vi "FlowPopup.vi"(11 "Path":path) -> ()   [LabVIEW 2013, in "main.lvlib"]
uses:
  main.lvlib
panel:
  out "Max amplitude 2":dbl
  out "Descending 2":dbl
  out "Ascending 2":dbl
  out "Max amplitude":dbl
  out "Descending":dbl
  out "Ascending":dbl
  in  "Cancel Button":bool
  out "RedGraph":T1(graph)
  out "BlueGraph":T1(graph)
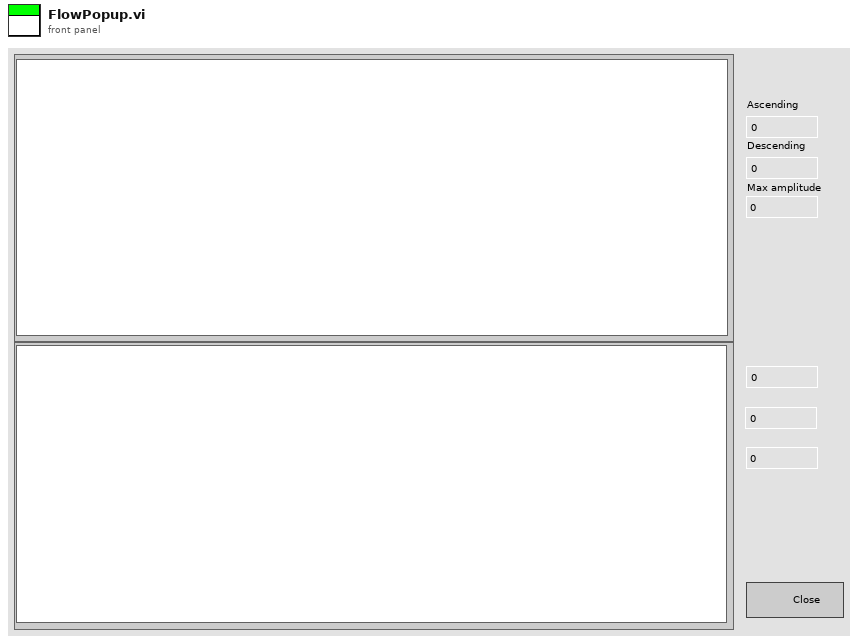
[diagram p1: front panel]
types:
  T1 = cluster{"Array out":dbl[], "Best Linear Fit":dbl[]}[]
  T2 = cluster{dbl[], "Best Linear Fit":dbl[], "slope":dbl, dbl[], "Best Linear Fit":dbl[], "slope":dbl}
  T3 = cluster{dbl[], "Best Linear Fit":dbl[], "slope":dbl}
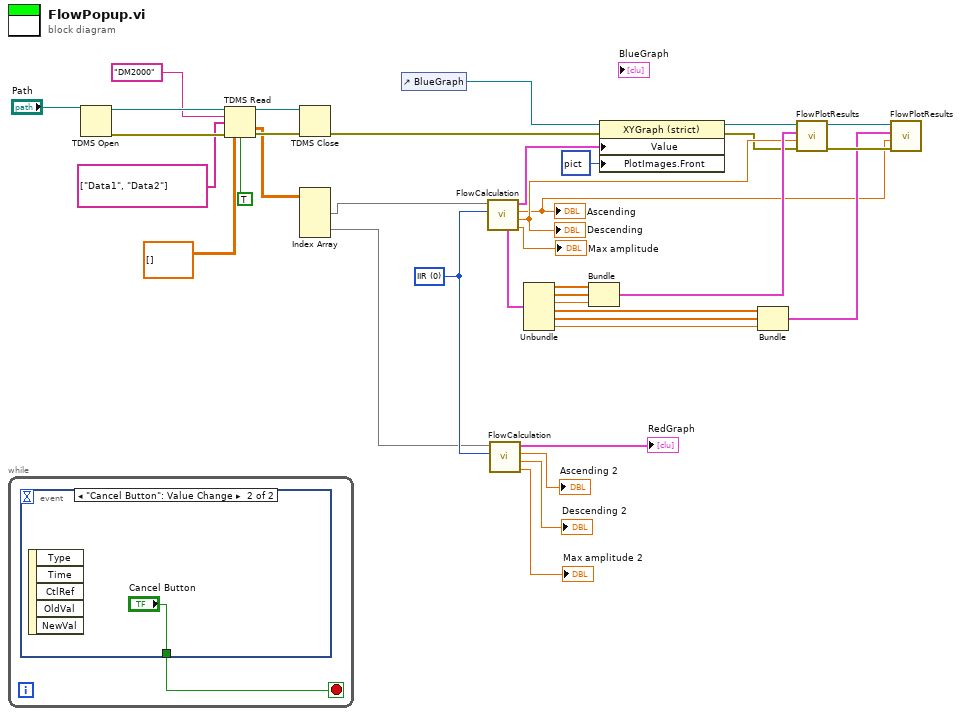
[diagram p0: block diagram]
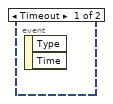
[diagram p2: hidden frame]
diagram:
  w36 = u16 0 items=["IIR", "Butterworth", "None"] ("Filter")
  n1 = while {
    stop <- w38 stop-if-true
    n2 = event shown="[1] \"Cancel Button\": Value Change" {
      selector: _ -> [_ _]
      dyn-events: _ -> [_ _]
      timeout: _ -> [_ _]
      tunnel: [_ "Cancel Button"] -> w38
      event Timeout {
        n3 = event-data() -> ()  [unwired: 1 in, 2 out]
      }
      event "Cancel Button": Value Change {
        n4 = event-data() -> ()  [unwired: 1 in, 5 out]
      }
    }
  }
  n5 = TDMS Open(11:"Path") -> (0:w29:errorcluster, 3:w35:refnum<k34>)  [unwired: 6 in]
  n6 = TDMS Read(0:w35, 5:"DM2000" ("group name in"), 7:string[] ["Data1", "Data2"], 11:w29, 12:dbl[][] [], 13:TRUE ("return channels in file order? (F)")) -> (4:w31:refnum<k34>, 10:w26:dbl[][], 15:w30:errorcluster)  [unwired: 2 in, 3 out]
  n7 = TDMS Close(8:w30, 11:w31) -> (0:w11:errorcluster)  [unwired: 1 out]
  n8 = Index Array(array=w26) -> (element #1=w25:dbl[], element #2=w24:dbl[])  [unwired: 4 in]
  n9 = control-ref of="BlueGraph"() -> (w14:refnum<vi>)
  n10 = call "FlowCalculation.vi"("Filter"=w36, "X"=w25) -> ("Max amplitude"=→"Max amplitude":dbl, "Descending"=w10:dbl, "Ascending"=w3:dbl, "Flow Graph"=w13:T1, "Slopes Out"=w19:T2)  [unwired: 5 in]
  "Ascending" <- w3
  "Descending" <- w10
  n11 = call "FlowCalculation.vi"("Filter"=w36, "X"=w24) -> ("Max amplitude"=→"Max amplitude 2":dbl, "Descending"=→"Descending 2":dbl, "Ascending"=→"Ascending 2":dbl, "Flow Graph"=→"RedGraph":T1)  [unwired: 5 in, 1 out]
  n12 = Unbundle(w19) -> (w18:dbl[], "Best Linear Fit"=w17:dbl[], "slope"=w16:dbl, w7:dbl[], "Best Linear Fit"=w6:dbl[], "slope"=w5:dbl)
  n13 = Bundle(w18, "Best Linear Fit"=w17, "slope"=w16) -> (w15:T3)  [unwired: 1 in]
  n14 = property class="XYGraph (strict)"(reference=w14, error in=w11, "Value"=w13, "PlotImages.Front"=picture data[5B] ("Plot Images:Front")) -> (reference out=w12:refnum<vi>, error out=w2:errorcluster)
  n15 = Bundle(w7, "Best Linear Fit"=w6, "slope"=w5) -> (w4:T3)  [unwired: 1 in]
  n16 = call "FlowPlotResults.vi"("error in (no error)"=w2, "Text"=w10, "Cluster"=w15, "Graph"=w12) -> ("error out"=w8:errorcluster, "reference out"=w9:refnum<vi>)  [unwired: 6 in]
  n17 = call "FlowPlotResults.vi"("error in (no error)"=w8, "Text"=w3, "Cluster"=w4, "Graph"=w9) -> ()  [unwired: 6 in, 2 out]
